vi "RT.vi"() -> ()   [LabVIEW 2011]
doc: "This is the primary Real-Time VI."
uses:
  <vilib>/Platform/TimedLoop/XDataNode/timing_clust.ctl
  <vilib>/Platform/TimedLoop/XDataNode/nitl_modes.ctl
  <vilib>/Platform/TimedLoop/XDataNode/wakeup.ctl
  <vilib>/rvi/Analysis/host/Butterworth/config/Butterworth Filter Type.ctl
  <vilib>/rvi/Analysis/host/Butterworth/config/Butterworth Filter Order.ctl
  <vilib>/FPGAPlugInAG/sbRIO-9636/niLvFpga_Open_sbRIO-9636.vi
  <vilib>/rvi/interface/common/dynamic/niFpgaDynamicAddResources.vi
  <vilib>/FPGAPlugInAG/Dynamic/niLvFpga_Reset_Dynamic.vi
  <vilib>/FPGAPlugInAG/Dynamic/niLvFpga_Run_Dynamic.vi
  <vilib>/Utility/error.llb/Error Cluster From Error Code.vi
  <vilib>/rvi/errors/niLvFpgaAdjustHostInterfaceError.vi
  <vilib>/FPGAPlugInAG/Dynamic/niLvFpga_Close_Dynamic.vi
  <vilib>/rvi/Analysis/host/Butterworth/config/BwScaledCoefficients.vi
  <vilib>/Platform/TimedLoop/XDataNode/XDataNode.xnode
  <vilib>/rvi/interface/nirviOpenFPGA/nirviOpenFPGA.xnode
  FPGA Bitfiles/TreadmillControl_FPGATarget_Exercise2_CF30559D.lvbitx
  FPGA/FPGA.vi
  <vilib>/rvi/interface/nirviMethod/nirviMethod.xnode
  <vilib>/rvi/interface/nirviReadWriteControl/nirviReadWriteControl.xnode
  <vilib>/rvi/interface/nirviCloseFPGA/nirviCloseFPGA.xnode
  <vilib>/rvi/Analysis/host/Butterworth/XNode/ButterworthCoefficients.xnode
  <vilib>/rvi/Analysis/host/Public/NI_FpgaMspHost.lvlib
  NiFpgaLv.dll
  <vilib>/rvi/interface/Simulation/niFpgaSimulationCallBeginRW.vi
  <vilib>/Platform/TimedLoop/XDataNode/XDNodeRunTimeDep.lvlib
panel:
  in  "Gain":dbl
  out "error out 2":errorcluster
  out "z out":sgl
  in  "PositionControl":bool
  in  "PID gains":T1={"proportional gain (Kc)"=1.0, "integral gain (Kc*Ts/Ti)"=0.015625, "derivative gain (Kc*Td/Ts)"=0.0}
  in  "PeriodHysteresis":fxp<+,23,4>=0.5
  in  "PeriodThreshold":fxp<+/-,24,5>=2.0
  in  "DeadCount":u32=30000
  out "PIDSetpoint":fxp<+/-,16,18>
  out "SpeedCommand":fxp<+/-,20,5>
  in  "ManualCommand":dbl
  in  "CommandCutoffFreq":dbl=100.0
  in  "UsePID":bool
  in  "ControlType":enum16{"Manual", "Potentiometer", "Sine"}(ring)
  in  "SineOffset":dbl
  in  "SinePeriod":dbl=100.0
  in  "SineAmplitude":dbl=1.0
  in  "SpeedCutoffFreq":dbl=100.0
  out "error out":errorcluster
  in  "Stop":bool
  in  "DriveEnable":bool
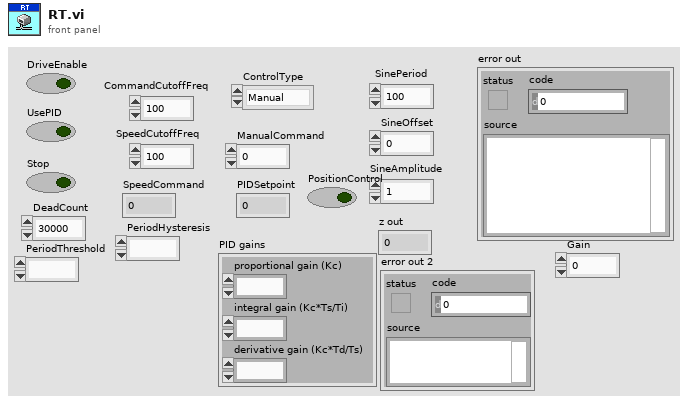
[diagram p1: front panel]
types:
  T1 = cluster{"proportional gain (Kc)":fxp<+/-,16,8>, "integral gain (Kc*Ts/Ti)":fxp<+/-,16,8>, "derivative gain (Kc*Td/Ts)":fxp<+/-,16,8>}
  T2 = typedef "XDNodeRunTimeDep.lvlib/timing_clust.ctl" = cluster{"Expected End [f-1]":u64, "Actual End [f-1]":u64, "Finished Late? [f-1]":bool, "Expected End [i-1]":u64, "Actual End [i-1]":u64, "Finished Late? [i-1]":bool, "Expected Start [i]":u64, "Actual Start [i]":u64, "Expected Start [f]":u64, "Actual Start [f]":u64, "Source Name":string, "Structure Name":string, "Period":i64, "Deadline":i64, "Offset":i64, "Start":i64, "Priority":i32, "Timeout":i32, "Mode":T3, "Wakeup Reason":T4, "Error":errorcluster, "Source Type":string, "Secondary Source Type":string, "Global End Time":u64, "Global Start Time":u64, "Frame Duration":u64, "Iteration Duration":u64, "Assigned CPU":i32, "I/O Scan Engine Mode":u32}
  T3 = typedef "XDNodeRunTimeDep.lvlib/nitl_modes.ctl" = enum32{"No Change", "Process missed periods, maintain original phase", "Discard missed periods, maintain original phase", "Process missed periods, ignore original phase", "Discard missed periods, ignore original phase"}
  T4 = typedef "XDNodeRunTimeDep.lvlib/wakeup.ctl" = enum32{"Normal", "Aborted", "Asynchronous wakeup", "Timing source error", "Timed loop error", "Timeout"}
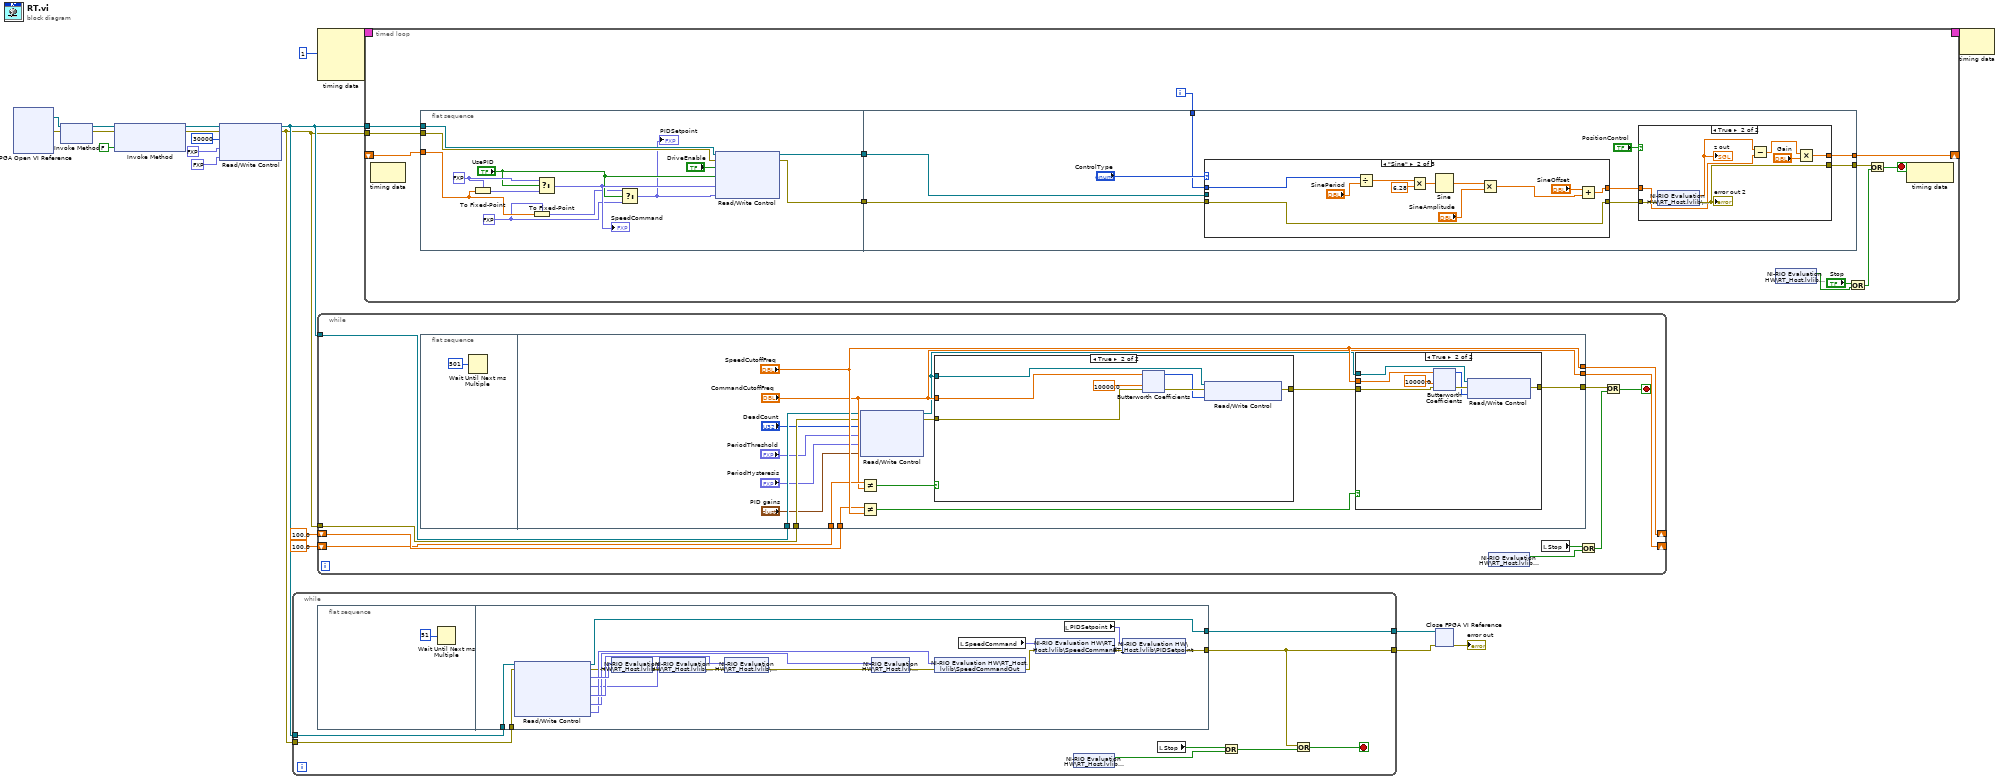
[diagram p0: block diagram]
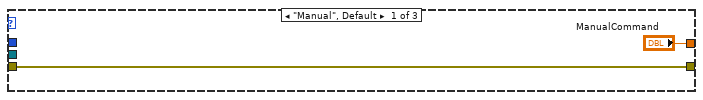
[diagram p5: hidden frame]
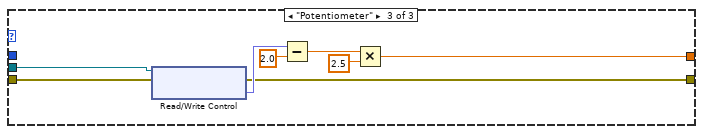
[diagram p6: hidden frame]
diagram:
  n1 = xnode "FPGA Open VI Reference"() -> ("FPGA VI Reference Out"=w20:refnum<k20>, "error out"=w19:errorcluster)  [unwired: 2 in]
  n2 = xnode "Invoke Method"("FPGA VI Reference In"=w20, "error in"=w19) -> ("FPGA VI Reference Out"=w18:refnum<k20>, "error out"=w17:errorcluster)
  n3 = xnode "Invoke Method"("FPGA VI Reference In"=w18, "error in"=w17, "Wait Until Done (F)"=FALSE) -> ("FPGA VI Reference Out"=w7:refnum<k20>, "error out"=w6:errorcluster)
  n4 = xnode "Read/Write Control"("FPGA VI Reference In"=w7, "error in"=w6, "DeadCount"=u32 30000, "PeriodThreshold"=fxp<+/-,24,5> 2.0, "PeriodThreshold"=fxp<+/-,24,5> 0.5) -> ("FPGA VI Reference Out"=w5:refnum<k20>, "error out"=w4:errorcluster)
  n5 = while {
    tunnel: w4 -> [w28]
    tunnel: w5 -> [w27]
    tunnel: [w22] -> w12
    tunnel: [w21] -> w11
    stop <- w23 stop-if-true
    n6 = flat-sequence {
      tunnel: w28 -> [w47]
      tunnel: w27 -> [w46]
      tunnel: [w31] -> w21
      tunnel: [w37] -> w22
      frame #0 {
        n7 = Wait Until Next ms Multiple(millisecond multiple=u32 51) -> ()  [unwired: 1 out]
      }
      frame #1 {
        n8 = xnode "Read/Write Control"("FPGA VI Reference In"=w46, "error in"=w47) -> ("FPGA VI Reference Out"=w37:refnum<k20>, "error out"=w36:errorcluster, "RPM"=w45:fxp<+,32,16>, "Speed"=w30:fxp<+/-,33,18>, "Accel"=w44:fxp<+/-,33,18>, "Jerk"=w43:fxp<+/-,37,22>, "SpeedCommandOut"=w39:fxp<+/-,23,8>)
        n9 = shared-variable "NI-RIO Evaluation HW\\RT_Host.lvlib\\RPM"(w45, error in=w36) -> (error out=w42:errorcluster)
        n10 = shared-variable "NI-RIO Evaluation HW\\RT_Host.lvlib\\Speed"(w30, error in=w42) -> (error out=w41:errorcluster)
        n11 = shared-variable "NI-RIO Evaluation HW\\RT_Host.lvlib\\Accel"(w44, error in=w41) -> (error out=w40:errorcluster)
        n12 = shared-variable "NI-RIO Evaluation HW\\RT_Host.lvlib\\Jerk"(w43, error in=w40) -> (error out=w38:errorcluster)
        n13 = shared-variable "NI-RIO Evaluation HW\\RT_Host.lvlib\\SpeedCommandOut"(w39, error in=w38) -> (error out=w35:errorcluster)
        n14 = local read "SpeedCommand"() -> (w34:fxp<+/-,20,5>)
        n15 = shared-variable "NI-RIO Evaluation HW\\RT_Host.lvlib\\SpeedCommand"(w34, error in=w35) -> (error out=w32:errorcluster)
        n16 = local read "PIDSetpoint"() -> (w33:fxp<+/-,16,18>)
        n17 = shared-variable "NI-RIO Evaluation HW\\RT_Host.lvlib\\PIDSetpoint"(w33, error in=w32) -> (error out=w31:errorcluster)
      }
    }
    n18 = shared-variable "NI-RIO Evaluation HW\\RT_Host.lvlib\\Stop"() -> (w26:bool)  [unwired: 1 in, 1 out]
    n19 = local read "Stop"() -> (w24:bool)
    n20 = Or(x=w24, y=w26) -> (x .or. y?=w25:bool)
    n21 = Or(x=w21, y=w25) -> (x .or. y?=w23:bool)
  }
  n22 = node-c288(i64 1 ("Period")) -> (w14:T2)  [unwired: 3 in]
  n23 = while {
    tunnel: w4 -> [w58]
    shift-right: [w52] -> _
    shift-left: 100.0 ("SpeedCutoffFreq") -> [w50]
    shift-right: [w51] -> _
    shift-left: 100.0 ("CommandCutoffFreq") -> [w49]
    tunnel: w5 -> [w48]
    stop <- w53 stop-if-true
    n24 = flat-sequence {
      tunnel: w58 -> [w65]
      tunnel: [w74] -> w54
      tunnel: ["SpeedCutoffFreq"] -> w52
      tunnel: ["CommandCutoffFreq"] -> w51
      tunnel: w50 -> [w72]
      tunnel: w49 -> [w71]
      tunnel: w48 -> [w67]
      frame #0 {
        n25 = Wait Until Next ms Multiple(millisecond multiple=u32 501) -> ()  [unwired: 1 out]
      }
      frame #1 {
        n26 = xnode "Read/Write Control"("FPGA VI Reference In"=w67, "error in"=w65, "DeadCount"="DeadCount", "PeriodThreshold"="PeriodThreshold", "PeriodHysteresis"="PeriodHysteresis", "PID gains"="PID gains") -> ("FPGA VI Reference Out"=w66:refnum<k20>, "error out"=w64:errorcluster)
        n27 = Not Equal?(x=w71, y="CommandCutoffFreq") -> (x != y?=w69:bool)
        n28 = Not Equal?(x=w72, y="SpeedCutoffFreq") -> (x != y?=w68:bool)
        n29 = case shown="True" w69 {
          tunnel: w64 -> [w91 w98]
          tunnel: [w91 w94] -> w75
          tunnel: "CommandCutoffFreq" -> [_ w97]
          tunnel: w66 -> [_ w92]
          frame False {
          }
          frame True {
            n30 = xnode "Butterworth Coefficients"("cutoff frequency (Hz)"=w97, "sample rate (S/s)"=10000.0, "error in (no error)"=w98) -> ("scaled coefficients"=w93:i32[], "error out"=w95:errorcluster)
            n31 = xnode "Read/Write Control"("FPGA VI Reference In"=w92, "error in"=w95, "CommandFilterCoeff"=w93) -> ("error out"=w94:errorcluster)  [unwired: 1 out]
          }
        }
        n32 = case shown="True" w68 {
          tunnel: w75 -> [w76 w83]
          tunnel: [w76 w79] -> w74
          tunnel: "SpeedCutoffFreq" -> [_ w82]
          tunnel: w66 -> [_ w78]
          frame False {
          }
          frame True {
            n33 = xnode "Butterworth Coefficients"("cutoff frequency (Hz)"=w82, "sample rate (S/s)"=10000.0, "error in (no error)"=w83) -> ("scaled coefficients"=w77:i32[], "error out"=w80:errorcluster)
            n34 = xnode "Read/Write Control"("FPGA VI Reference In"=w78, "error in"=w80, "SpeedFilterCoeff"=w77) -> ("error out"=w79:errorcluster)  [unwired: 1 out]
          }
        }
      }
    }
    n35 = shared-variable "NI-RIO Evaluation HW\\RT_Host.lvlib\\Stop"() -> (w55:bool)  [unwired: 1 in, 1 out]
    n36 = local read "Stop"() -> (w57:bool)
    n37 = Or(x=w57, y=w55) -> (x .or. y?=w56:bool)
    n38 = Or(x=w54, y=w56) -> (x .or. y?=w53:bool)
  }
  n39 = timed-loop {
    tunnel: w5 -> [w113]
    tunnel: w4 -> [w112]
    timing: w14 -> [_]
    timing-out: [_] -> w13
    shift-right: [w106] -> _
    shift-left: _ -> [w107]
    i -> [w111]
    stop <- w117 stop-if-true
    n40 = node-c288() -> ()  [unwired: 1 in, 1 out]
    n41 = flat-sequence {
      tunnel: w113 -> [w132]
      tunnel: w112 -> [w131]
      tunnel: [w129] -> w110
      tunnel: [w128] -> w109
      tunnel: w107 -> [w127]
      tunnel: w111 -> [w140]
      tunnel: w110 -> [w139]
      tunnel: w109 -> [w138]
      tunnel: [w133] -> w108
      tunnel: [w135] -> w106
      frame #0 {
        w120 = fxp<+/-,16,18> 0.0 ("PIDSetpoint")
        w126 = fxp<+/-,20,5> 0.0 ("SpeedCommand")
        n42 = To Fixed-Point(fixed-point type=w126, number=w127) -> (fixed-point=w125:fxp<+/-,20,5>)
        n43 = To Fixed-Point(fixed-point type=w120, number=w127) -> (fixed-point=w122:fxp<+/-,16,18>)
        n44 = Select(t=w126, s="UsePID", f=w125) -> (s? t:f=w124:fxp<+/-,20,5>)
        "SpeedCommand" <- w124
        n45 = Select(t=w122, s="UsePID", f=w120) -> (s? t:f=w121:fxp<+/-,16,18>)
        "PIDSetpoint" <- w121
        n46 = xnode "Read/Write Control"("FPGA VI Reference In"=w132, "error in"=w131, "DriveEnable"="DriveEnable", "UsePID"="UsePID", "SpeedCommand"=w124, "PIDSetpoint"=w121) -> ("FPGA VI Reference Out"=w129:refnum<k20>, "error out"=w128:errorcluster)
      }
      frame #1 {
        n47 = case shown="\"Sine\"" "ControlType" {
          tunnel: w140 -> [_ w155 _]
          tunnel: w139 -> [_ _ w167]
          tunnel: w138 -> [w152 w154 w166]
          tunnel: [w152 w154 w165] -> w134
          tunnel: ["ManualCommand" w153 w164] -> w136
          frame "Manual", Default {
          }
          frame "Sine" {
            n48 = Divide(x=w155, y="SinePeriod") -> (x/y=w159:dbl)
            n49 = Multiply(x=w159, y=6.28) -> (x*y=w160:dbl)
            n50 = Sine(x=w160) -> (sin(x)=w156:dbl)
            n51 = Multiply(x=w156, y="SineAmplitude") -> (x*y=w162:dbl)
            n52 = Add(x="SineOffset", y=w162) -> (x+y=w153:dbl)
          }
          frame "Potentiometer" {
            n53 = xnode "Read/Write Control"("FPGA VI Reference In"=w167, "error in"=w166) -> ("error out"=w165:errorcluster, "Potentiometer"=w170:fxp<+/-,24,5>)  [unwired: 1 out]
            n54 = Subtract(x=w170, y=2.0 ("sample rate (S/s)")) -> (x-y=w171:dbl)
            n55 = Multiply(x=w171, y=2.5 ("sample rate (S/s)")) -> (x*y=w164:dbl)
          }
        }
        n56 = case shown="True" "PositionControl" {
          tunnel: w136 -> [w143 w146]
          tunnel: [w143 w145] -> w135
          tunnel: w134 -> [w142 w148]
          tunnel: [w142 w147] -> w133
          frame False {
          }
          frame True {
            n57 = shared-variable "NI-RIO Evaluation HW\\RT_Host.lvlib\\z out"(error in=w148) -> (w149:sgl, error out=w147:errorcluster)
            "z out" <- w149
            "error out 2" <- w147
            n58 = Subtract(x=w149, y=w146) -> (x-y=w150:dbl)
            n59 = Multiply(x=w150, y="Gain") -> (x*y=w145:dbl)
          }
        }
      }
    }
    n60 = shared-variable "NI-RIO Evaluation HW\\RT_Host.lvlib\\Stop"() -> (w115:bool)  [unwired: 1 in, 1 out]
    n61 = Or(x="Stop", y=w115) -> (x .or. y?=w116:bool)
    n62 = Or(x=w108, y=w116) -> (x .or. y?=w117:bool)
    n63 = node-c288() -> ()  [unwired: 1 in, 1 out]
  }
  n64 = xnode "Close FPGA VI Reference"("FPGA VI Reference In"=w12, "error in"=w11) -> ("error out"=→"error out":errorcluster)
  n65 = node-c288(w13) -> ()  [unwired: 1 out]
